vi "Format Command to md.vi"(8 "error in (no error)":errorcluster, 10 "firstRow?":bool, 11 "line":string) -> (0 "error out":errorcluster, 2 "lua row":string, 3 ".md table row":string)   [LabVIEW 2019, in "LINXx.lvlib"]
doc: "Formats specific command information for documentation table"
uses:
  LINXx.lvlib
  <vilib>/regexp/Match Regular Expression.xnode
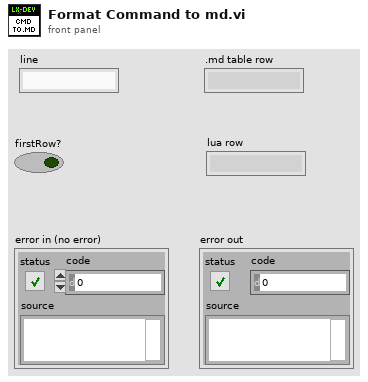
[diagram p1: front panel]
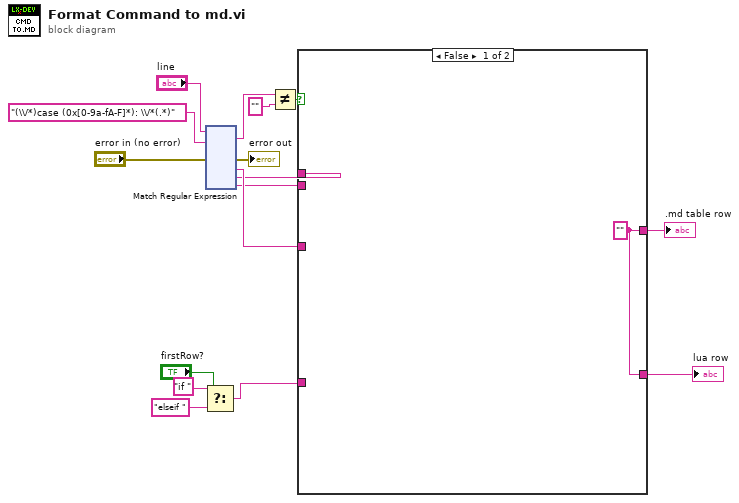
[diagram p0: block diagram]
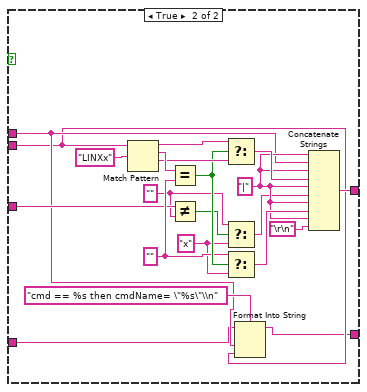
[diagram p2: hidden frame]
diagram:
  n1 = Select(t="if " ("y"), s="firstRow?", f="elseif ") -> (s? t:f=w4:string)
  n2 = xnode "Match Regular Expression"("input string"="line", "regular expression"="(\\/*)case (0x[0-9a-fA-F]*): \\/*(.*)", "error in"="error in (no error)") -> ("whole match"=w15:string, "error out"=→"error out":errorcluster, "submatch 1"=w11:string, "submatch 2"=w8:string, "submatch 3"=w9:string)  [unwired: 3 in, 3 out]
  n3 = Not Equal?(x=w15, y="") -> (x != y?=w16:bool)
  n4 = case shown="False" w16 {
    tunnel: w8 -> [_ w21]
    tunnel: w9 -> [_ w20]
    tunnel: [w17 w29] -> w10
    tunnel: w11 -> [_ w26]
    tunnel: [w17 w19] -> w5
    tunnel: w4 -> [_ w18]
    frame False {
      w17 = ""
    }
    frame True {
      w25 = "" ("y")
      w24 = "x" ("f")
      w32 = "" ("y")
      w30 = "|" ("string")
      n5 = Match Pattern(string=w20, regular expression="LINXx") -> (before substring=w36:string, match substring=w37:string, after substring=w35:string)  [unwired: 1 in, 1 out]
      n6 = Equal?(x=w37, y=w32) -> (x = y?=w33:bool)
      n7 = Not Equal?(x=w26, y=w25) -> (x != y?=w27:bool)
      n8 = Select(t=w36, s=w33, f=w35) -> (s? t:f=w34:string)
      n9 = Select(t=w25, s=w27, f=w24) -> (s? t:f=w23:string)
      n10 = Select(t=w32, s=w33, f=w24) -> (s? t:f=w31:string)
      n11 = Format Into String(format string="cmd == %s then cmdName= \"%s\"\\n", initial string=w18, w21, w20) -> (resulting string=w19:string)  [unwired: 1 in, 1 out]
      n12 = Concatenate Strings(w30, w21, w30, w34, w30, w23, w30, w31, w30, "\r\n") -> (w29:string)
    }
  }
  ".md table row" <- w10
  "lua row" <- w5
